vi "CheckForError-TMP.vi"(0 "Main Path":path) -> (1 "Array of Folders":path[](array[path]), 2 "PRAMMS-CommVRN":refnum<visa-resource-name>, 3 "Array of Files":path[](array[path]), 4 "Master Dir":path, 6 "Bundle-Meteo":T1={"cRIO address"="0.0.0.0", "Port Number"=0, "cRIO_commID"=refnum, "Cx"=FALSE}, 8 "This VI's Path":path, 10 "term":string, 11 "Go on ?":bool, 12 "Array of Baud Rates":u32[](array[numeric]), 13 "TCS-CommVRN":refnum<visa-resource-name>, 14 "Array of VISA refnum":refnum<visa-resource-name>[](array[refnum]), 15 "Serial":bool[](array[boolean]))   [LabVIEW 2011]
uses:
  Globals.vi
  <vilib>/Utility/config.llb/Read Key (U32).vi
  <vilib>/Utility/config.llb/Read Key (String).vi
  <vilib>/Instr/_visa.llb/VISA Configure Serial Port (Instr).vi
  <vilib>/Utility/config.llb/Read Key (Path).vi
  <vilib>/Utility/config.llb/NI_LVConfig.lvlib
panel:
  out "PRAMMS":bool
  out "ActiveDummy":bool
  out "TCS":bool
  out "TCP Error":errorcluster
  out "standard output":string
  out "standard error":string
  out "concatenated string":string
  out "Nettoyage":bool
  in  "restart":bool
  out "error out":errorcluster
  in  "cancel":bool
  in  "ignore":bool
  out "IDL":bool
  out "wget":bool
  out "Ports Series":bool
  out "SubVIs":bool
  out "config error out":errorcluster
  out "Camera":bool
  out "Starry Night":bool
  out "Configuration":bool
  out "Arborescence":bool
  # "Version sans GUI de ErrorCheck.vi  Vérifie :\n    - Existence des chemins/fichiers nécessaire\n    - Communication avec les différents périphériques\n    - Lien ActiveX avec Starry Night\n    - Vérifie la communication avec la station météo\n    - Vérifie l'état de la face avant des VIs utilisés\n    - Compatibilité des versions installées\n    - Vérifie la disponibilité des applications (wget, IDL)"
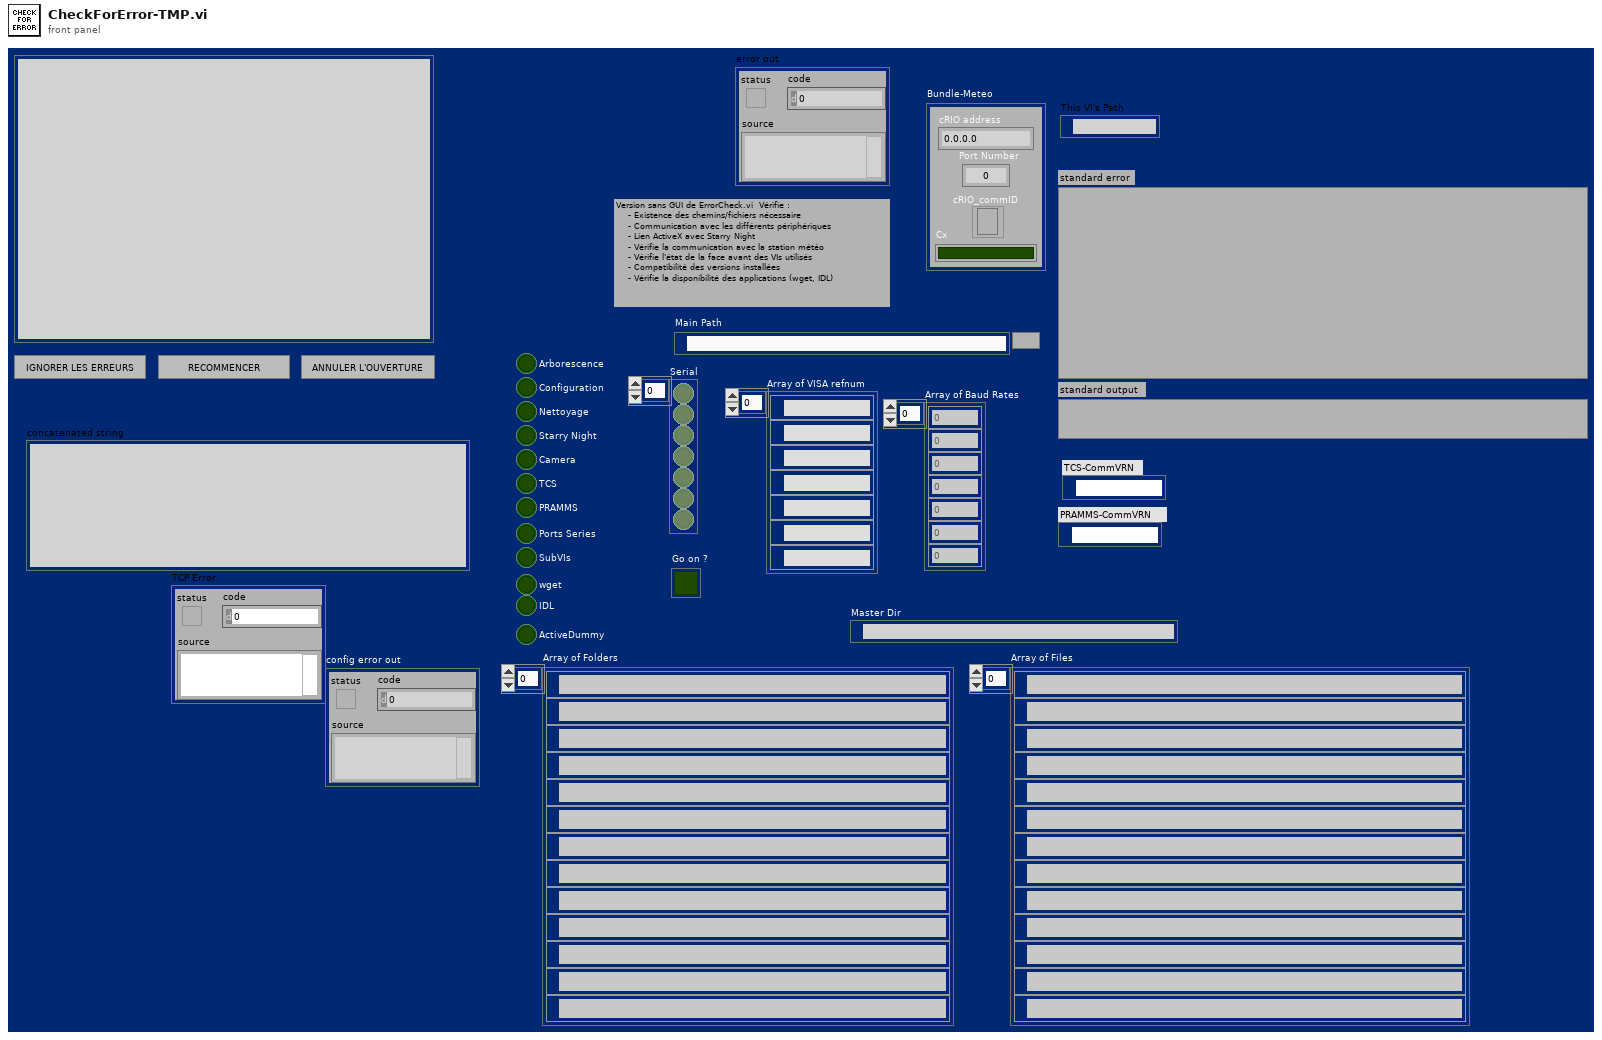
[diagram p1: front panel]
types:
  T1 = cluster{"cRIO address":string, "Port Number":u16, "cRIO_commID":refnum<k5>, "Cx":bool}
  T2 = enum8{"Enabled", "Disabled", "Disabled and Grayed Out"}
  T3 = typedef "NI_LVConfig.lvlib/Config Data RefNum.ctl" = refnum<k1>
  T4 = cluster{"value":string, u16, "connection ID":refnum<k5>, bool}
  T5 = enum16{"Left Button", "Center Button", "Right Button", "Window Close"}
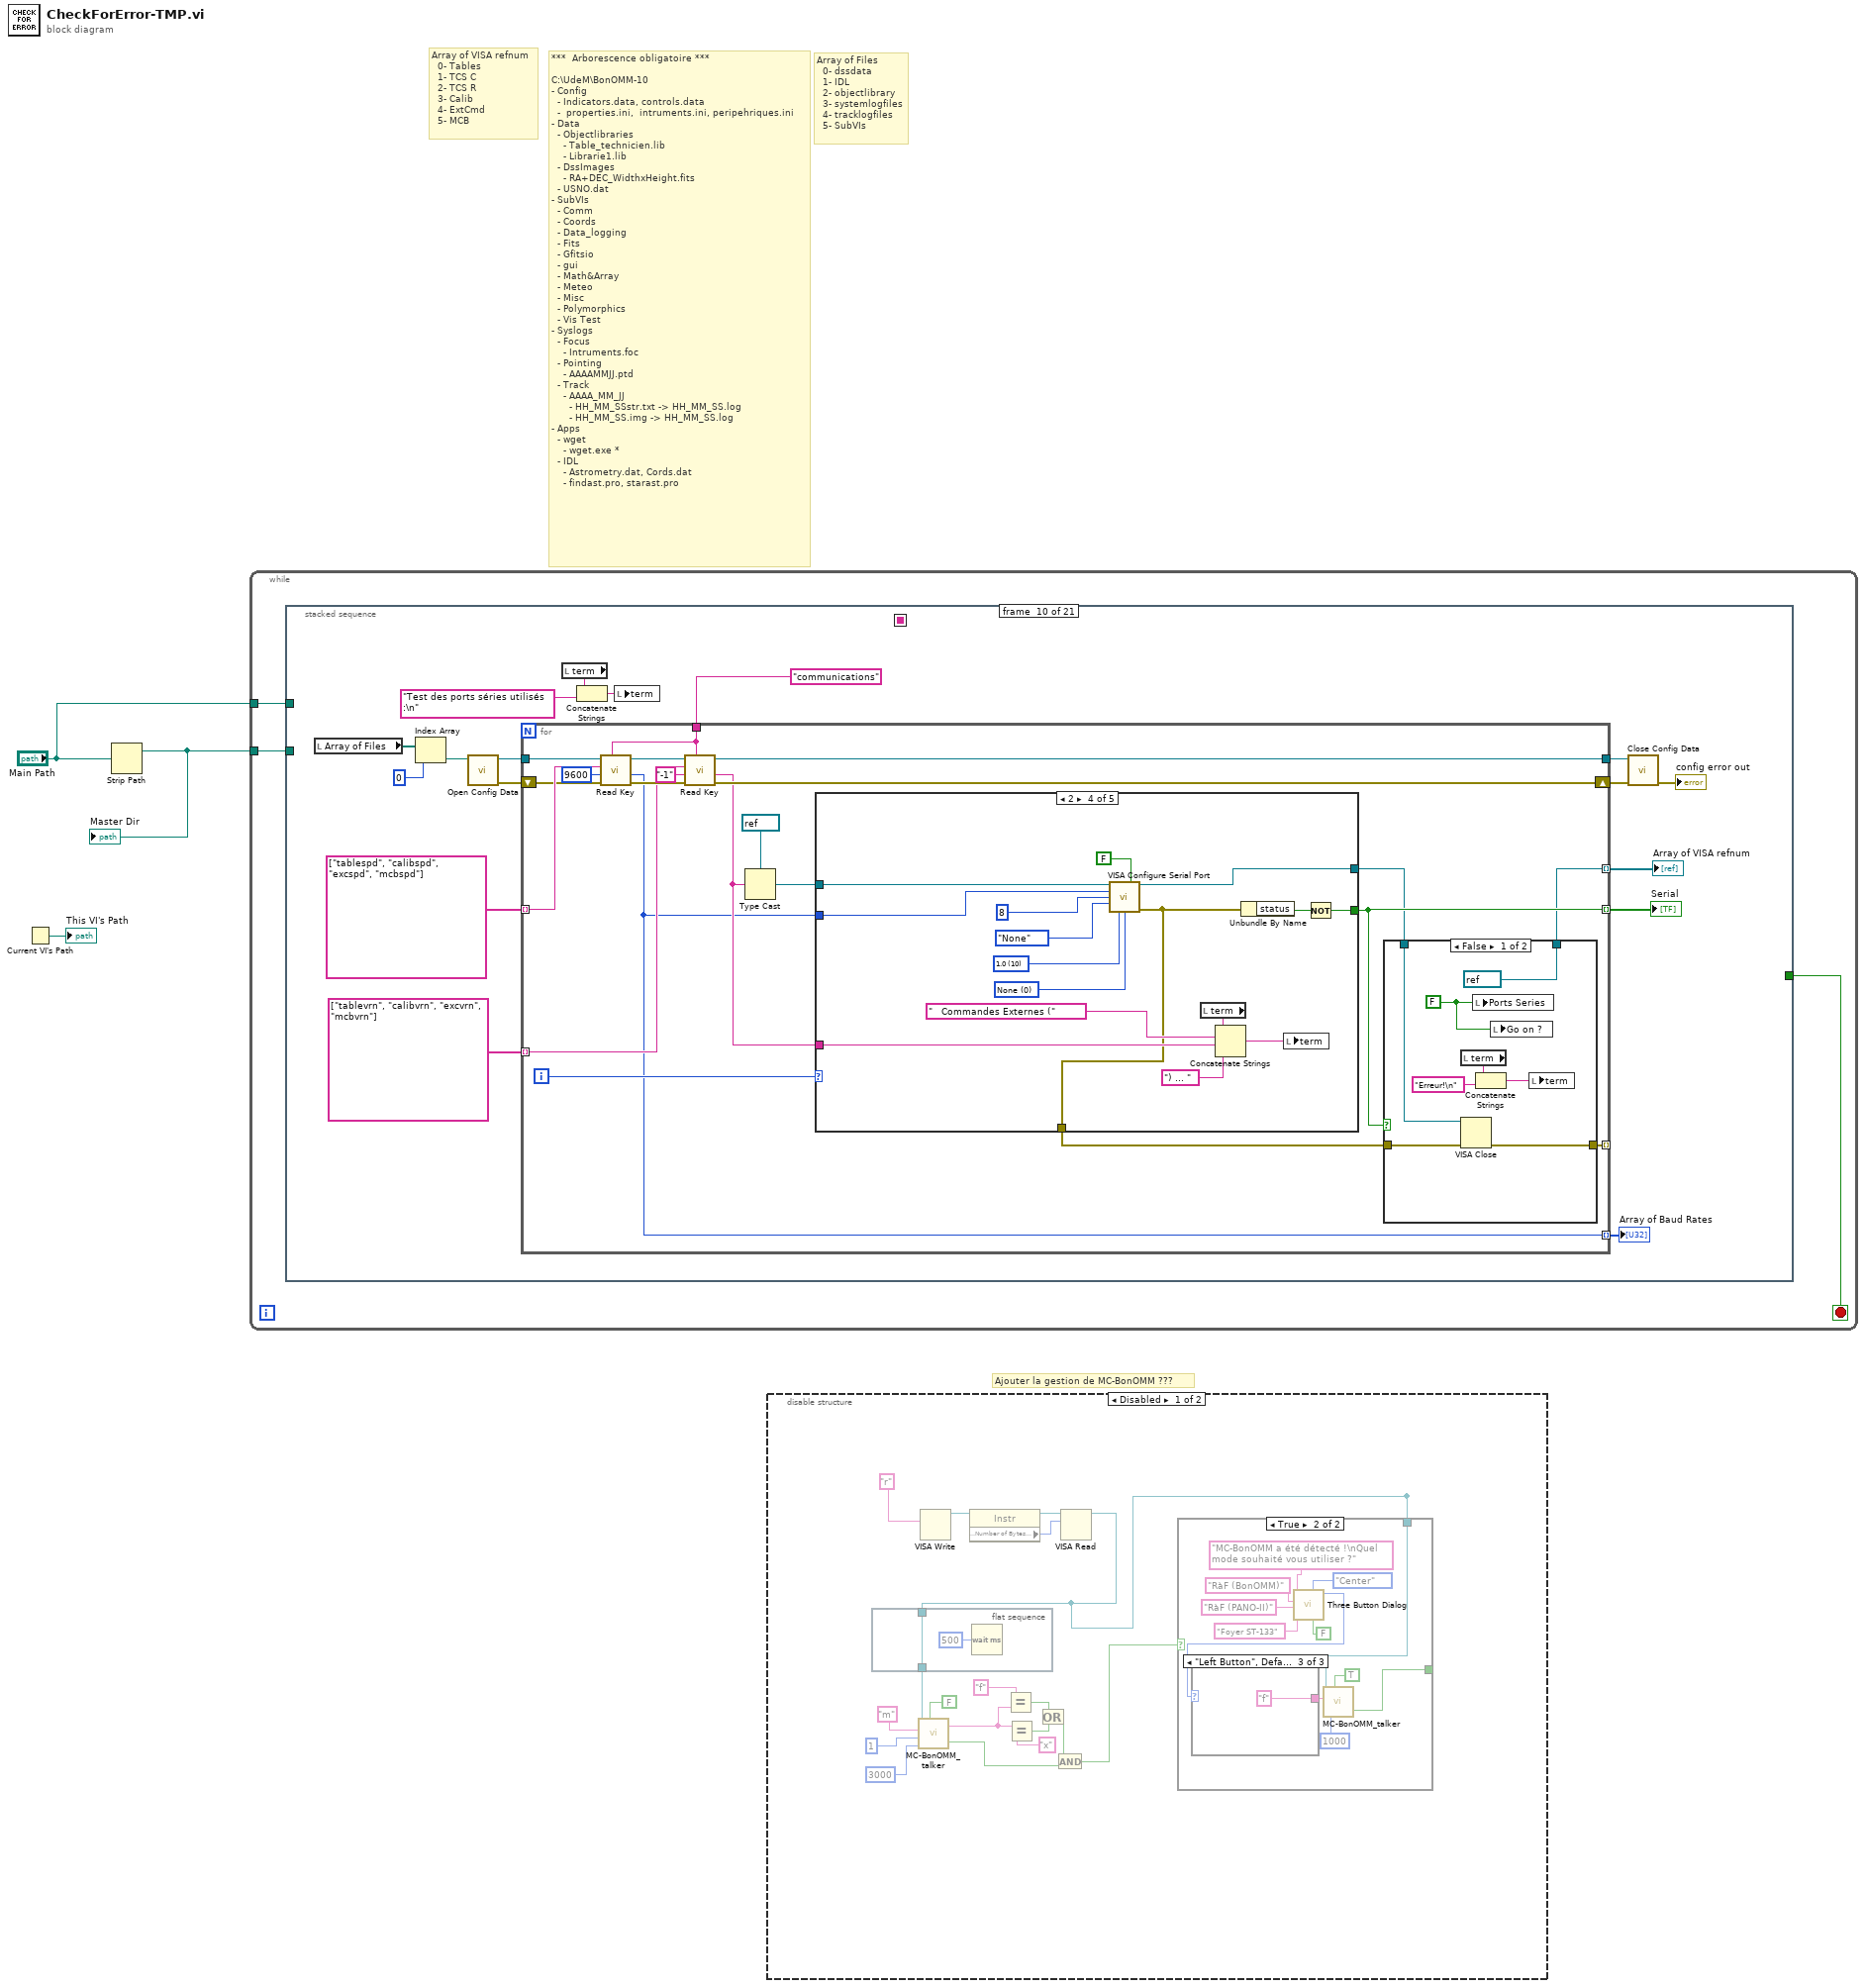
[diagram p0: block diagram]
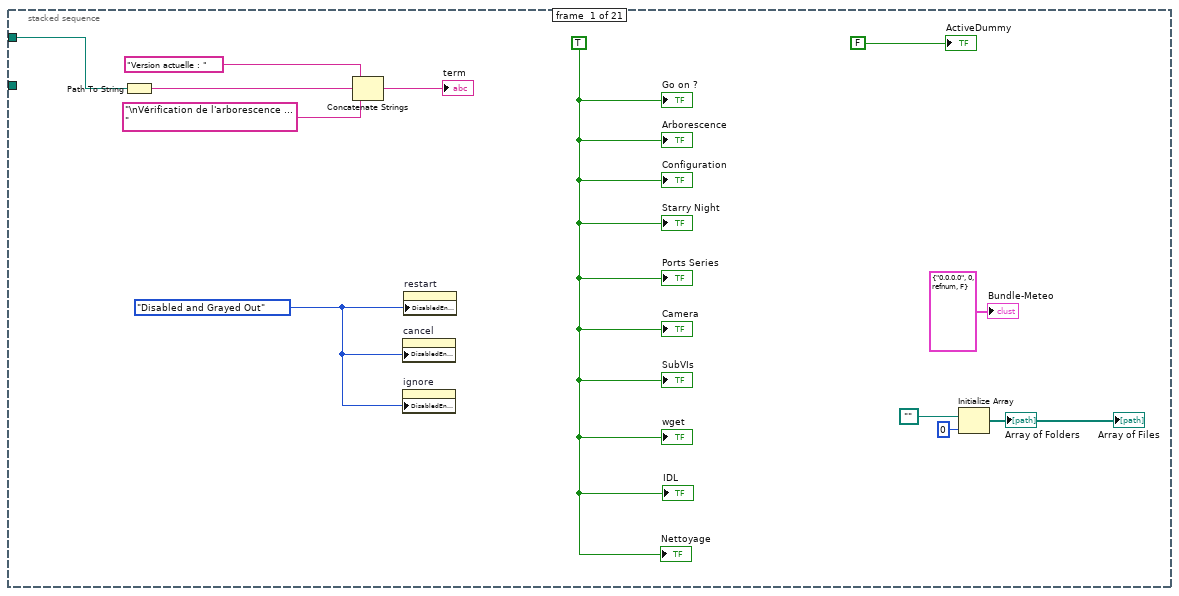
[diagram p2: hidden frame]
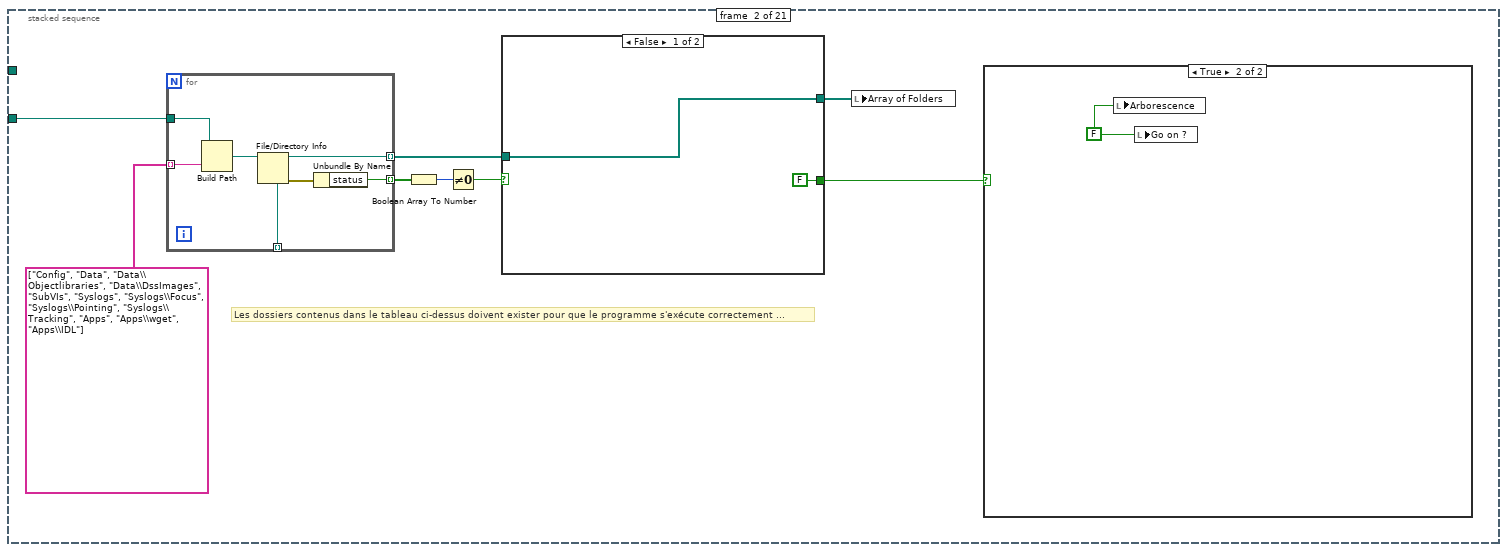
[diagram p3: hidden frame]
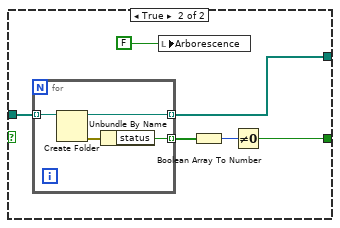
[diagram p5: hidden frame]
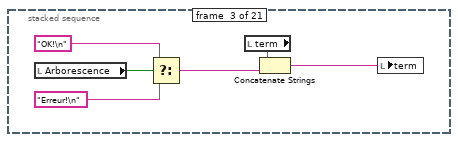
[diagram p6: hidden frame]
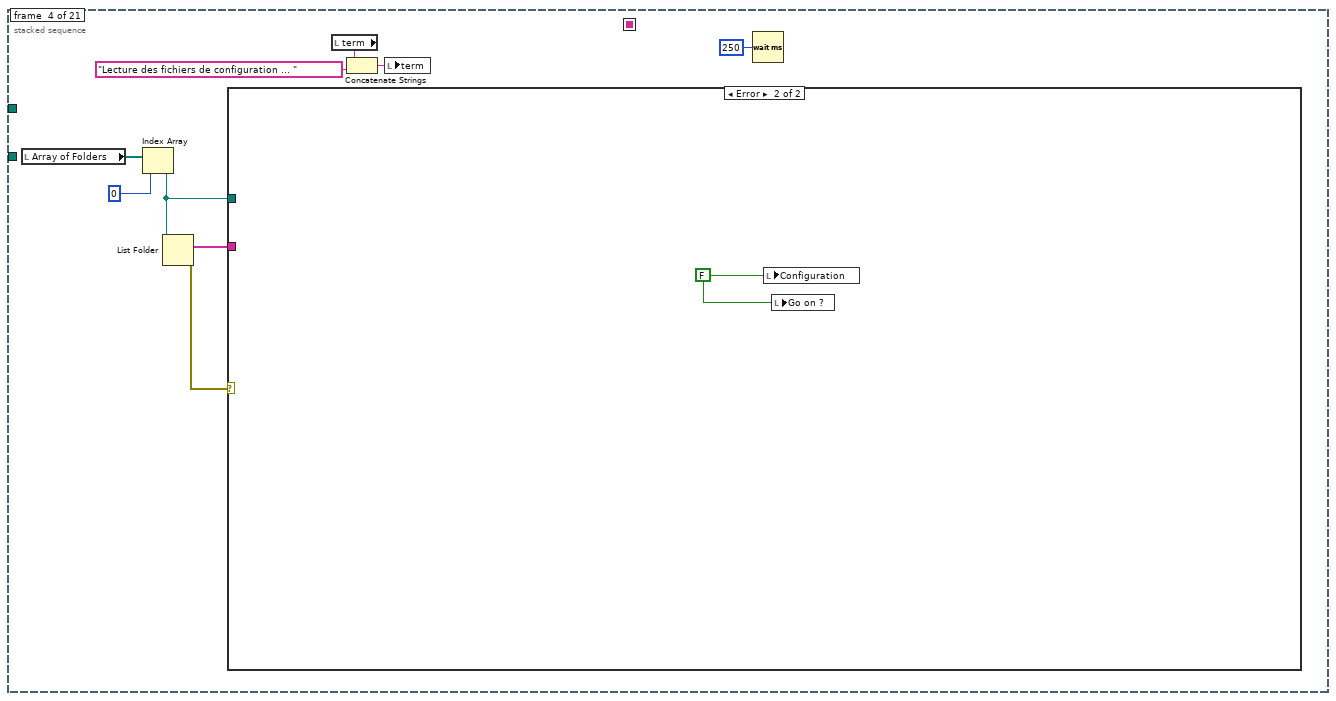
[diagram p7: hidden frame]
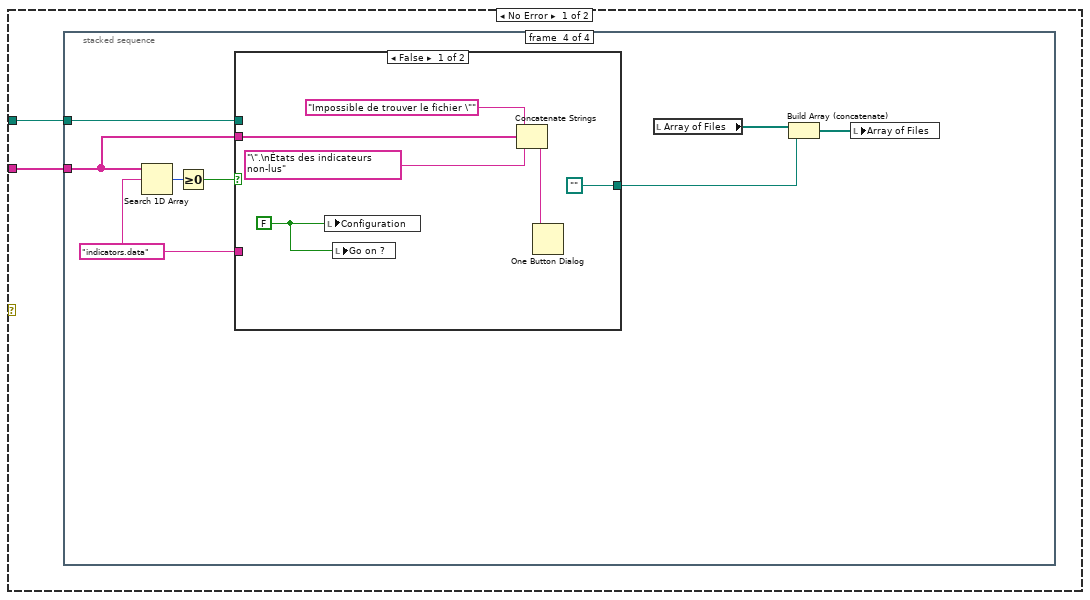
[diagram p8: hidden frame]
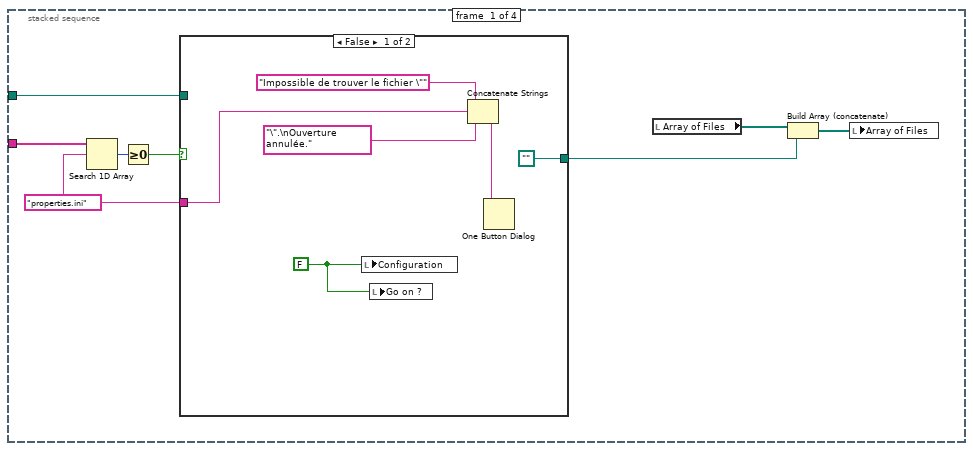
[diagram p9: hidden frame]
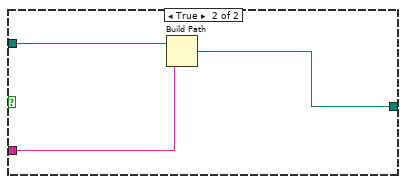
[diagram p10: hidden frame]
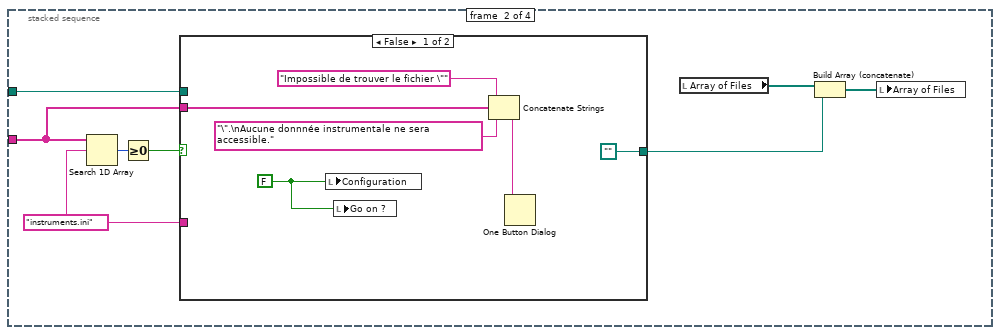
[diagram p11: hidden frame]
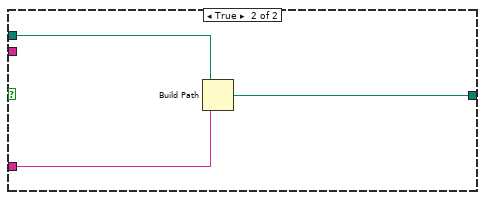
[diagram p12: hidden frame]
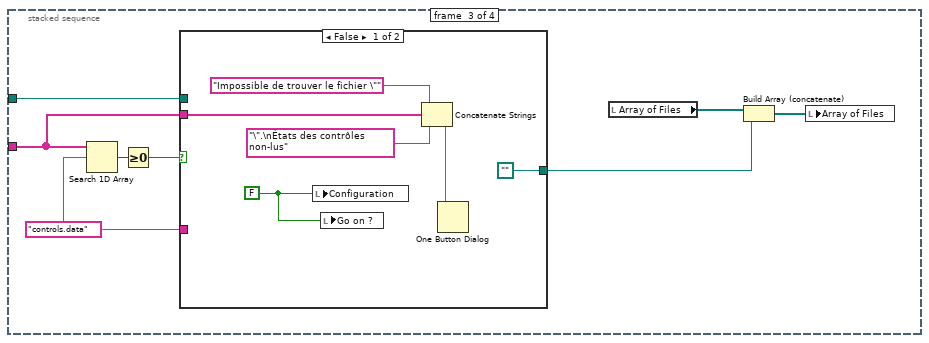
[diagram p13: hidden frame]
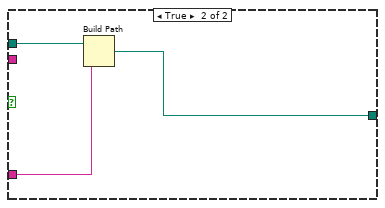
[diagram p14: hidden frame]
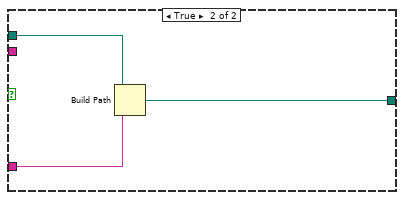
[diagram p15: hidden frame]
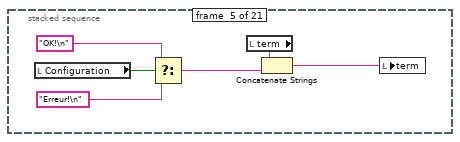
[diagram p16: hidden frame]
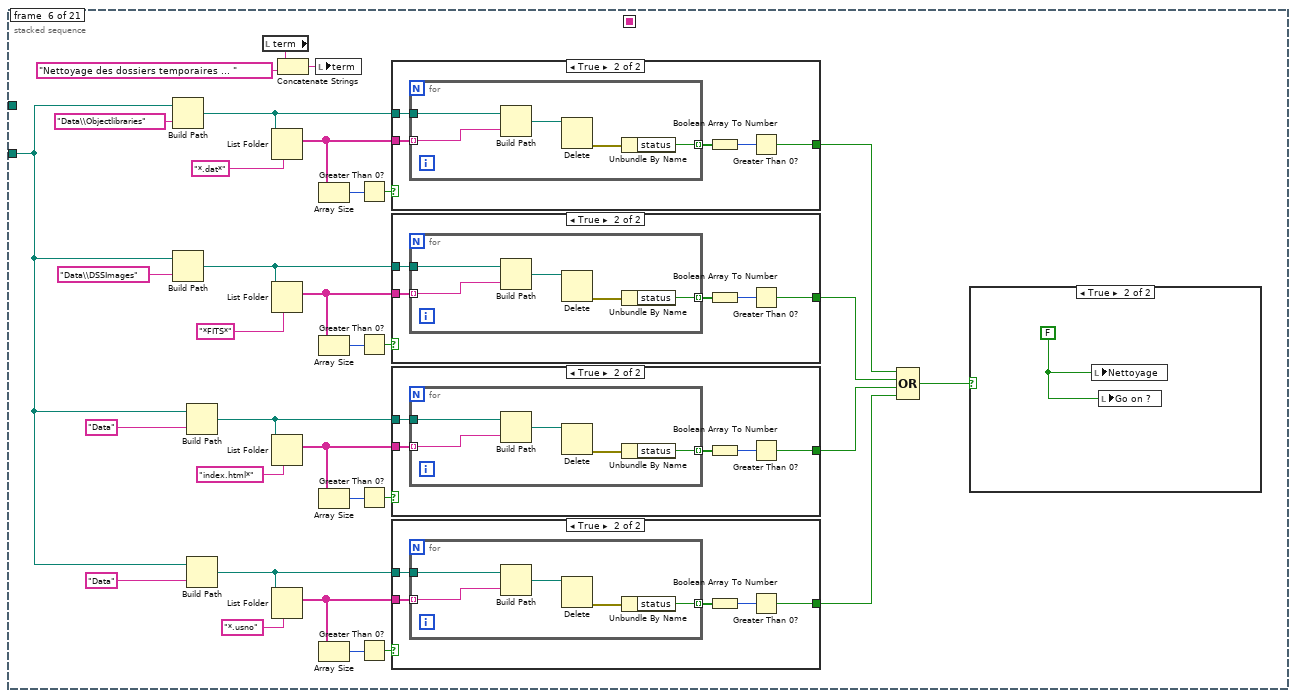
[diagram p17: hidden frame]
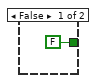
[diagram p18: hidden frame]
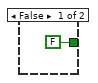
[diagram p19: hidden frame]
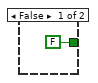
[diagram p20: hidden frame]
diagram:
  # "Array of Files\n  0- dssdata\n  1- IDL\n  2- objectlibrary\n  3- systemlogfiles\n  4- tracklogfiles\n  5- SubVIs"
  # "***  Arborescence obligatoire ***\n\nC:\\UdeM\\BonOMM-10\n-\tConfig\n  -\tIndicators.data, controls.data\n  -\t properties.ini,  intruments.ini, peripehriques.ini\n-\tData\n  -\tObjectlibraries\n    -\tTable_technicien.lib\n    -\tLibrarie1.lib\n  -\tDssImages\n    -\tRA+DEC_WidthxHeight.fits\n  -\tUSNO.dat\n-\tSubVIs\n  -\tComm\n  -\tCoords\n  -\tData_logging\n  -\tFits\n  -\tGfitsio\n  -\tgui\n  -\tMath&Array\n  -\tMeteo\n  -\tMisc\n  -\tPolymorphics\n  -\tVis Test\n-\tSyslogs\n  -\tFocus\n    -\tIntruments.foc\n  -\tPointing\n    -\tAAAAMMJJ.ptd\n  -\tTrack\n    -\tAAAA_MM_JJ\n      -\tHH_MM_SSstr.txt -> HH_MM_SS.log\n      -\tHH_MM_SS.img -> HH_MM_SS.log\n-\tApps\n  -\twget\n    -\twget.exe *\n  -\tIDL\n    -\tAstrometry.dat, Cords.dat\n    -\tfindast.pro, starast.pro"
  # "Array of VISA refnum\n  0- Tables\n  1- TCS C\n  2- TCS R\n  3- Calib\n  4- ExtCmd\n  5- MCB"
  # "Ajouter la gestion de MC-BonOMM ???"
  n1 = Current VI's Path() -> (path=→"This VI's Path":path)
  n2 = Strip Path(path="Main Path") -> (stripped path=w3:path)  [unwired: 1 out]
  "Master Dir" <- w3
  n3 = while {
    tunnel: w3 -> [w6]
    tunnel: "Main Path" -> [w5]
    stop <- w4 stop-if-true
    n4 = stacked-sequence {
      seq-local: [_ _ _ _ _ _ _ _ _ _ _ _ _ _ _ _ _ _ _ w594 _] -> [_ _ _ _ _ _ _ _ _ _ _ _ _ _ _ _ _ _ _ _ w630]
      tunnel: w6 -> [_ w25 _ _ _ w139 _ _ _ _ _ _ _ _ _ _ _ _ _ _ _]
      tunnel: w5 -> [w14 _ _ _ _ _ _ _ _ _ _ _ _ _ _ _ _ _ _ _ _]
      tunnel: [_ _ _ _ _ _ _ _ _ _ _ _ _ _ _ _ _ _ _ w595 _] -> w4
      frame #0 {
        w9 = T2."Disabled and Grayed Out" ("Disabled")
        w8 = TRUE ("Arborescence")
        n5 = Path To String(path=w14) -> (string=w18:string)
        n6 = Concatenate Strings("Version actuelle : ", w18, "\nVérification de l'arborescence ... ") -> (→"term":string)
        n7 = property on="cancel" class="Bool"("DisabledEnum"=w9) -> ()  [unwired: 2 in, 2 out]
        n8 = property on="ignore" class="Bool"("DisabledEnum"=w9) -> ()  [unwired: 2 in, 2 out]
        n9 = property on="restart" class="Bool"("DisabledEnum"=w9) -> ()  [unwired: 2 in, 2 out]
        n10 = Initialize Array(path "" ("path dup"), 0 ("dimension size")) -> (→"Array of Folders" →"Array of Files":path[])
        "Arborescence" <- w8
        "Go on ?" <- w8
        "Configuration" <- w8
        "Starry Night" <- w8
        "Camera" <- w8
        "SubVIs" <- w8
        "Ports Series" <- w8
        "wget" <- w8
        "IDL" <- w8
        "Bundle-Meteo" <- T1 {"cRIO address"="0.0.0.0", "Port Number"=0, "cRIO_commID"=refnum, "Cx"=FALSE} ("Bundle-Meteo")
        "Nettoyage" <- w8
        "ActiveDummy" <- FALSE ("Arborescence")
      }
      frame #1 {
        # "Les dossiers contenus dans le tableau ci-dessus doivent exister pour que le programme s'exécute correctement ..."
        n11 = for {
          tunnel: string[] ["Config", "Data", "Data\\Objectlibraries", "Data\\DssImages", "SubVIs", "Syslogs", "Syslogs\\Focus", "Syslogs\\Pointing", "Syslogs\\Tracking", "Apps", "Apps\\wget", "Apps\\IDL"] -> [w45] mode=indexing
          tunnel: w25 -> [w46]
          tunnel: [w43] -> w21 mode=indexing
          tunnel: [w42] -> _ mode=indexing
          tunnel: [w40] -> w24 mode=indexing
          n12 = Build Path(base path=w46, name or relative path=w45) -> (appended path=w44:path)
          n13 = File/Directory Info(path=w44) -> (path out=w43:path, error out=w41:errorcluster, resolved path=w42:path)  [unwired: 1 in, 4 out]
          n14 = Unbundle By Name(w41) -> ("status"=w40:bool)
        }
        n15 = Boolean Array To Number(Boolean array=w24) -> (number=w23:u32)
        n16 = Not Equal To 0?(x=w23) -> (x != 0?=w22:bool)
        n17 = case shown="False" w22 {
          tunnel: w21 -> [w28 w35]
          tunnel: [FALSE w32] -> w20
          tunnel: [w28 w31] -> w19
          frame False {
          }
          frame True {
            n18 = for {
              tunnel: w35 -> [w39] mode=indexing
              tunnel: [w37] -> w33 mode=indexing
              tunnel: [w36] -> w31 mode=indexing
              n19 = Create Folder(path (use dialog)=w39) -> (created path=w36:path, error out=w38:errorcluster)  [unwired: 2 in, 1 out]
              n20 = Unbundle By Name(w38) -> ("status"=w37:bool)
            }
            n21 = local write "Arborescence"(FALSE) -> ()
            n22 = Boolean Array To Number(Boolean array=w33) -> (number=w34:u32)
            n23 = Not Equal To 0?(x=w34) -> (x != 0?=w32:bool)
          }
        }
        n24 = local write "Array of Folders"(w19) -> ()
        n25 = case shown="True" w20 {
          frame False {
          }
          frame True {
            w27 = FALSE
            n26 = local write "Arborescence"(w27) -> ()
            n27 = local write "Go on ?"(w27) -> ()
          }
        }
      }
      frame #2 {
        n28 = local read "Arborescence"() -> (w49:bool)
        n29 = Select(t="OK!\n" ("string"), s=w49, f="Erreur!\n" ("string")) -> (s? t:f=w50:string)
        n30 = local read "term"() -> (w51:string)
        n31 = Concatenate Strings(w51, w50) -> (w52:string)
        n32 = local write "term"(w52) -> ()
      }
      frame #3 {
        n33 = local read "Array of Folders"() -> (w55:path[])
        n34 = Index Array(array=w55, index=0) -> (element=w53:path)
        n35 = List Folder(path=w53) -> (filenames=w58:string[], error out=w56:errorcluster)  [unwired: 3 in, 2 out]
        n36 = case shown="Error" w56 {
          tunnel: w58 -> [w63 _]
          tunnel: w53 -> [w62 _]
          frame No Error {
            n37 = stacked-sequence {
              tunnel: w63 -> [w69 w86 w103 w120]
              tunnel: w62 -> [w66 w84 w102 w119]
              frame #0 {
                w65 = "properties.ini"
                n38 = Search 1D Array(1D array=w69, element=w65) -> (index of element=w71:i32)  [unwired: 1 in]
                n39 = Greater Or Equal To 0?(x=w71) -> (x >= 0?=w70:bool)
                n40 = case shown="False" w70 {
                  tunnel: w66 -> [_ w80]
                  tunnel: w65 -> [w73 w79]
                  tunnel: [path "" w78] -> w64
                  frame False {
                    w74 = FALSE ("Configuration")
                    n41 = local write "Configuration"(w74) -> ()
                    n42 = local write "Go on ?"(w74) -> ()
                    n43 = Concatenate Strings("Impossible de trouver le fichier \"", w73, "\".\nOuverture annulée.") -> (w75:string)
                    n44 = One Button Dialog(message=w75) -> ()  [unwired: 1 in, 1 out]
                  }
                  frame True {
                    n45 = Build Path(base path=w80, name or relative path=w79) -> (appended path=w78:path)
                  }
                }
                n46 = local read "Array of Files"() -> (w68:path[])
                n47 = Build Array (concatenate)(w68, w64) -> (w67:path[])
                n48 = local write "Array of Files"(w67) -> ()
              }
              frame #1 {
                w85 = "instruments.ini"
                n49 = Search 1D Array(1D array=w86, element=w85) -> (index of element=w88:i32)  [unwired: 1 in]
                n50 = Greater Or Equal To 0?(x=w88) -> (x >= 0?=w87:bool)
                n51 = case shown="False" w87 {
                  tunnel: w86 -> [w92 _]
                  tunnel: w85 -> [_ w97]
                  tunnel: w84 -> [_ w96]
                  tunnel: [path "" w95] -> w81
                  frame False {
                    w90 = FALSE ("Configuration")
                    n52 = local write "Configuration"(w90) -> ()
                    n53 = local write "Go on ?"(w90) -> ()
                    n54 = Concatenate Strings("Impossible de trouver le fichier \"", w92, "\".\nAucune donnnée instrumentale ne sera accessible.") -> (w91:string)
                    n55 = One Button Dialog(message=w91) -> ()  [unwired: 1 in, 1 out]
                  }
                  frame True {
                    n56 = Build Path(base path=w96, name or relative path=w97) -> (appended path=w95:path)
                  }
                }
                n57 = local read "Array of Files"() -> (w83:path[])
                n58 = Build Array (concatenate)(w83, w81) -> (w82:path[])
                n59 = local write "Array of Files"(w82) -> ()
              }
              frame #2 {
                w101 = "controls.data"
                n60 = Search 1D Array(1D array=w103, element=w101) -> (index of element=w105:i32)  [unwired: 1 in]
                n61 = Greater Or Equal To 0?(x=w105) -> (x >= 0?=w104:bool)
                n62 = case shown="False" w104 {
                  tunnel: w103 -> [w109 _]
                  tunnel: w102 -> [_ w114]
                  tunnel: w101 -> [_ w113]
                  tunnel: [path "" w112] -> w98
                  frame False {
                    w107 = FALSE ("Configuration")
                    n63 = local write "Configuration"(w107) -> ()
                    n64 = local write "Go on ?"(w107) -> ()
                    n65 = Concatenate Strings("Impossible de trouver le fichier \"", w109, "\".\nÉtats des contrôles non-lus") -> (w108:string)
                    n66 = One Button Dialog(message=w108) -> ()  [unwired: 1 in, 1 out]
                  }
                  frame True {
                    n67 = Build Path(base path=w114, name or relative path=w113) -> (appended path=w112:path)
                  }
                }
                n68 = local read "Array of Files"() -> (w100:path[])
                n69 = Build Array (concatenate)(w100, w98) -> (w99:path[])
                n70 = local write "Array of Files"(w99) -> ()
              }
              frame #3 {
                w118 = "indicators.data"
                n71 = Search 1D Array(1D array=w120, element=w118) -> (index of element=w122:i32)  [unwired: 1 in]
                n72 = Greater Or Equal To 0?(x=w122) -> (x >= 0?=w121:bool)
                n73 = case shown="False" w121 {
                  tunnel: w120 -> [w126 _]
                  tunnel: w119 -> [_ w131]
                  tunnel: w118 -> [_ w130]
                  tunnel: [path "" w129] -> w115
                  frame False {
                    w124 = FALSE ("Configuration")
                    n74 = local write "Configuration"(w124) -> ()
                    n75 = local write "Go on ?"(w124) -> ()
                    n76 = Concatenate Strings("Impossible de trouver le fichier \"", w126, "\".\nÉtats des indicateurs non-lus") -> (w125:string)
                    n77 = One Button Dialog(message=w125) -> ()  [unwired: 1 in, 1 out]
                  }
                  frame True {
                    n78 = Build Path(base path=w131, name or relative path=w130) -> (appended path=w129:path)
                  }
                }
                n79 = local read "Array of Files"() -> (w117:path[])
                n80 = Build Array (concatenate)(w117, w115) -> (w116:path[])
                n81 = local write "Array of Files"(w116) -> ()
              }
            }
          }
          frame Error {
            w132 = FALSE ("Configuration")
            n82 = local write "Configuration"(w132) -> ()
            n83 = local write "Go on ?"(w132) -> ()
          }
        }
        n84 = local read "term"() -> (w60:string)
        n85 = Concatenate Strings(w60, "Lecture des fichiers de configuration ... " ("string")) -> (w61:string)
        n86 = local write "term"(w61) -> ()
        n87 = Wait (ms)(milliseconds to wait=u32 250) -> ()  [unwired: 1 out]
      }
      frame #4 {
        n88 = local read "Configuration"() -> (w135:bool)
        n89 = Select(t="OK!\n" ("string"), s=w135, f="Erreur!\n" ("string")) -> (s? t:f=w136:string)
        n90 = local read "term"() -> (w137:string)
        n91 = Concatenate Strings(w137, w136) -> (w138:string)
        n92 = local write "term"(w138) -> ()
      }
      frame #5 {
        n93 = Build Path(base path=w139, name or relative path="Data\\Objectlibraries") -> (appended path=w164:path)
        n94 = Build Path(base path=w139, name or relative path="Data\\DSSImages") -> (appended path=w162:path)
        n95 = Build Path(base path=w139, name or relative path="Data") -> (appended path=w148:path)
        n96 = Build Path(base path=w139, name or relative path="Data") -> (appended path=w145:path)
        n97 = local read "term"() -> (w170:string)
        n98 = List Folder(path=w164, pattern="*.dat*") -> (filenames=w166:string[])  [unwired: 2 in, 3 out]
        n99 = List Folder(path=w162, pattern="*FITS*") -> (filenames=w160:string[])  [unwired: 2 in, 3 out]
        n100 = List Folder(path=w148, pattern="index.html*") -> (filenames=w150:string[])  [unwired: 2 in, 3 out]
        n101 = List Folder(path=w145, pattern="*.usno") -> (filenames=w144:string[])  [unwired: 2 in, 3 out]
        n102 = Concatenate Strings(w170, "Nettoyage des dossiers temporaires ... " ("string")) -> (w171:string)
        n103 = local write "term"(w171) -> ()
        n104 = Array Size(array=w166) -> (size(s)=w167:i32)
        n105 = Array Size(array=w160) -> (size(s)=w159:i32)
        n106 = Array Size(array=w150) -> (size(s)=w151:i32)
        n107 = Array Size(array=w144) -> (size(s)=w143:i32)
        n108 = Greater Than 0?(x=w167) -> (x > 0?=w168:bool)
        n109 = Greater Than 0?(x=w159) -> (x > 0?=w158:bool)
        n110 = Greater Than 0?(x=w151) -> (x > 0?=w152:bool)
        n111 = Greater Than 0?(x=w143) -> (x > 0?=w142:bool)
        n112 = case shown="True" w168 {
          tunnel: w166 -> [_ w210]
          tunnel: w164 -> [_ w209]
          tunnel: [FALSE w206] -> w156
          frame False {
          }
          frame True {
            n113 = for {
              tunnel: w210 -> [w214] mode=indexing
              tunnel: w209 -> [w215]
              tunnel: [w211] -> w208 mode=indexing
              n114 = Build Path(base path=w215, name or relative path=w214) -> (appended path=w213:path)
              n115 = Delete(path (use dialog)=w213) -> (error out=w212:errorcluster)  [unwired: 4 in, 2 out]
              n116 = Unbundle By Name(w212) -> ("status"=w211:bool)
            }
            n117 = Boolean Array To Number(Boolean array=w208) -> (number=w207:u32)
            n118 = Greater Than 0?(x=w207) -> (x > 0?=w206:bool)
          }
        }
        n119 = case shown="True" w158 {
          tunnel: w160 -> [_ w199]
          tunnel: w162 -> [_ w198]
          tunnel: [FALSE w195] -> w155
          frame False {
          }
          frame True {
            n120 = for {
              tunnel: w199 -> [w203] mode=indexing
              tunnel: w198 -> [w204]
              tunnel: [w200] -> w197 mode=indexing
              n121 = Build Path(base path=w204, name or relative path=w203) -> (appended path=w202:path)
              n122 = Delete(path (use dialog)=w202) -> (error out=w201:errorcluster)  [unwired: 4 in, 2 out]
              n123 = Unbundle By Name(w201) -> ("status"=w200:bool)
            }
            n124 = Boolean Array To Number(Boolean array=w197) -> (number=w196:u32)
            n125 = Greater Than 0?(x=w196) -> (x > 0?=w195:bool)
          }
        }
        n126 = case shown="True" w152 {
          tunnel: w150 -> [_ w188]
          tunnel: w148 -> [_ w187]
          tunnel: [FALSE w184] -> w149
          frame False {
          }
          frame True {
            n127 = for {
              tunnel: w188 -> [w192] mode=indexing
              tunnel: w187 -> [w193]
              tunnel: [w189] -> w186 mode=indexing
              n128 = Build Path(base path=w193, name or relative path=w192) -> (appended path=w191:path)
              n129 = Delete(path (use dialog)=w191) -> (error out=w190:errorcluster)  [unwired: 4 in, 2 out]
              n130 = Unbundle By Name(w190) -> ("status"=w189:bool)
            }
            n131 = Boolean Array To Number(Boolean array=w186) -> (number=w185:u32)
            n132 = Greater Than 0?(x=w185) -> (x > 0?=w184:bool)
          }
        }
        n133 = case shown="True" w142 {
          tunnel: w144 -> [_ w177]
          tunnel: w145 -> [_ w176]
          tunnel: [FALSE w173] -> w140
          frame False {
          }
          frame True {
            n134 = for {
              tunnel: w177 -> [w181] mode=indexing
              tunnel: w176 -> [w182]
              tunnel: [w178] -> w175 mode=indexing
              n135 = Build Path(base path=w182, name or relative path=w181) -> (appended path=w180:path)
              n136 = Delete(path (use dialog)=w180) -> (error out=w179:errorcluster)  [unwired: 4 in, 2 out]
              n137 = Unbundle By Name(w179) -> ("status"=w178:bool)
            }
            n138 = Boolean Array To Number(Boolean array=w175) -> (number=w174:u32)
            n139 = Greater Than 0?(x=w174) -> (x > 0?=w173:bool)
          }
        }
        n140 = Compound Arithmetic op=OR(w156, w155, w149, w140) -> (w157:bool)
        n141 = case shown="True" w157 {
          frame False {
          }
          frame True {
            w216 = FALSE
            n142 = local write "Nettoyage"(w216) -> ()
            n143 = local write "Go on ?"(w216) -> ()
          }
        }
      }
      frame #6 {
        n144 = local read "Nettoyage"() -> (w219:bool)
        n145 = Select(t="OK!\n" ("string"), s=w219, f="Erreur!\n" ("string")) -> (s? t:f=w220:string)
        n146 = local read "term"() -> (w221:string)
        n147 = Concatenate Strings(w221, w220) -> (w222:string)
        n148 = local write "term"(w222) -> ()
      }
      frame #7 {
        n149 = local read "term"() -> (w229:string)
        n150 = Concatenate Strings(w229, "Test du lien ActiveX avec Starry Night ... " ("string")) -> (w230:string)
        n151 = local write "term"(w230) -> ()
        n152 = Automation Open(Automation Refnum=refnum<k7> refnum ("ScopeSim._Telescope")) -> (Automation Refnum=w223:refnum<k7>, error out=w226:errorcluster)  [unwired: 3 in]
        n153 = Unbundle By Name(w226) -> ("status"=w225:bool)
        n154 = case shown="True" w225 {
          tunnel: w223 -> [w233 _]
          tunnel: [w232 FALSE ("Connected")] -> w227
          frame False {
            n155 = property class="_Telescope"(reference=w233) -> (reference out=w231:refnum<k7>, "Connected"=w232:bool)  [unwired: 1 in, 1 out]
            n156 = Close Reference(reference=w231) -> ()  [unwired: 1 in, 1 out]
          }
          frame True {
          }
        }
        n157 = global write "Globals.vi" "ScopeSim._Telescope"(w223) -> ()
        n158 = case shown="True" w227 {
          frame False {
            w235 = FALSE
            n159 = local write "Starry Night"(w235) -> ()
            n160 = local write "Go on ?"(w235) -> ()
          }
          frame True {
          }
        }
      }
      frame #8 {
        n161 = local read "Starry Night"() -> (w236:bool)
        n162 = Select(t="OK!\n" ("string"), s=w236, f="Erreur!\n" ("string")) -> (s? t:f=w239:string)
        n163 = local read "term"() -> (w240:string)
        n164 = Concatenate Strings(w240, w239) -> (w241:string)
        n165 = local write "term"(w241) -> ()
      }
      frame #9 {
        n166 = local read "Array of Files"() -> (w244:path[])
        n167 = Index Array(array=w244, index=0) -> (element=w243:path)
        n168 = call <vilib>:"Open Config Data.vi"("configuration file path"=w243) -> ("error out"=w252:errorcluster, "refnum"=w254:T3)  [unwired: 8 in, 1 out]
        n169 = for {
          tunnel: string[] ["tablespd", "calibspd", "excspd", "mcbspd"] -> [w275] mode=indexing
          tunnel: string[] ["tablevrn", "calibvrn", "excvrn", "mcbvrn"] -> [w274] mode=indexing
          tunnel: "communications" -> [w267]
          tunnel: w254 -> [w277]
          tunnel: [w276] -> w253
          shift-right: [w272] -> w251
          shift-left: w252 -> [w273]
          tunnel: [w264] -> w247 mode=indexing
          tunnel: [w266] -> w246 mode=indexing
          tunnel: [w260] -> w245 mode=indexing
          tunnel: [w262] -> _ mode=indexing
          i -> [w268]
          n170 = call-poly <vilib>:"Read Key.vi"("section"=w267, "error in (no error)"=w273, "default value"=u32 9600, "key"=w275, "refnum"=w277) -> ("error out"=w278:errorcluster, "value"=w260:u32, "refnum out"=w279:T3)  [unwired: 3 in, 1 out]
          n171 = call-poly <vilib>:"Read Key.vi"("section"=w267, "error in (no error)"=w278, "default value"="-1", "key"=w274, "refnum"=w279) -> ("error out"=w272:errorcluster, "value"=w263:string, "refnum out"=w276:T3)  [unwired: 3 in, 1 out]
          n172 = Type Cast(type=refnum<visa-resource-name> "-1" ("Table VRN"), x=w263) -> (*(type *) &x=w261:refnum<visa-resource-name>)
          n173 = case shown="2" w268 {
            tunnel: w261 -> [_ w308 w317 w338 w354]
            tunnel: [refnum<visa-resource-name> "-1" ("Table VRN") w300 w329 w336 w352] -> w265
            tunnel: [FALSE ("ok ?") w304 w330 w348 w359] -> w266
            tunnel: w263 -> [_ w312 w324 w343 w360]
            tunnel: w260 -> [_ w302 w319 w337 w353]
            tunnel: [errorcluster {"status"=FALSE, "code"=0, "source"=""} ("error out") w297 w316 w335 w351] -> w259
            frame -1, Default {
              (unwired) "Bizzarerie ... " ("string")
            }
            frame 0 {
              n174 = control-ref of="ActiveDummy"() -> (w296:refnum<vi>)
              n175 = Equal?(x=refnum<visa-resource-name> "N/A" ("Table VRN"), y=w308) -> (x = y?=w306:bool)
              n176 = Select(t=refnum<visa-resource-name> "-1", s=w306, f=w308) -> (s? t:f=w303:refnum<visa-resource-name>)
              n177 = call "Newmark-Initialize.vi"("VISA resource name"=w303, "ActiveStages"=string[] ["AX", "AY", "AZ"], "baud rate"=w302, "Timeout"=u32 1000, "Bool Refnum"=w296) -> ("VISA resource name out"=w300:refnum<visa-resource-name>, "Error?"=w299:bool, "Error OUT"=w297:errorcluster)  [unwired: 8 in]
              n178 = Not(x=w306) -> (.not. x?=w307:bool)
              n179 = local read "term"() -> (w315:string)
              n180 = Concatenate Strings(w315, "   Table de guidage (" ("string"), w312, ") ... " ("string")) -> (w314:string)
              n181 = And(x=w299, y=w307) -> (x .and. y?=w305:bool)
              n182 = Not(x=w305) -> (.not. x?=w304:bool)
              n183 = local write "term"(w314) -> ()
            }
            frame 1 {
              w323 = u16 0 items=["None", "XON/XOFF", "RTS/CTS", "XON/XOFF & RTS/CTS", "DTR/DSR", "XON/XOFF & DTR/DSR"] ("flow control (0:none)")
              w322 = u16 10 items=["1.0"=10, "1.5"=15, "2.0"=20] ("stop bits (10: 1 bit)")
              n184 = call-poly "VISA Configure Serial Port"("VISA resource name"=w317, "baud rate (9600)"=w319, "data bits (8)"=u16 8, "parity (0:none)"=enum16{"None", "Odd", "Even", "Mark", "Space"}."None", "stop bits (10: 1 bit)"=w322, "flow control (0:none)"=w323) -> ("VISA resource name out"=w318:refnum<visa-resource-name>, "error out"=w316:errorcluster)  [unwired: 8 in]
              n185 = call "Controle_des_lampe.vi"("VISA resource name"=w318, "Status In"=bool[] [FALSE, FALSE, FALSE]) -> ("VISA resource name dup"=w329:refnum<visa-resource-name>, "Status Out"=w333:bool[])  [unwired: 1 out]
              n186 = local read "term"() -> (w328:string)
              n187 = Concatenate Strings(w328, "   Module de caibration (" ("string"), w324, ") ... " ("string")) -> (w327:string)
              n188 = Boolean Array To Number(Boolean array=w333) -> (number=w331:u32)
              n189 = Equal To 0?(x=w331) -> (x = 0?=w330:bool)
              n190 = local write "term"(w327) -> ()
            }
            frame 2 {
              w342 = u16 0 items=["None", "XON/XOFF", "RTS/CTS", "XON/XOFF & RTS/CTS", "DTR/DSR", "XON/XOFF & DTR/DSR"] ("flow control (0:none)")
              w341 = u16 10 items=["1.0"=10, "1.5"=15, "2.0"=20] ("stop bits (10: 1 bit)")
              n191 = call-poly "VISA Configure Serial Port"("VISA resource name"=w338, "Enable Termination\nChar (T)"=FALSE ("Enable Termination\nChar (T)"), "baud rate (9600)"=w337, "data bits (8)"=u16 8, "parity (0:none)"=enum16{"None", "Odd", "Even", "Mark", "Space"}."None", "stop bits (10: 1 bit)"=w341, "flow control (0:none)"=w342) -> ("VISA resource name out"=w336:refnum<visa-resource-name>, "error out"=w335:errorcluster)  [unwired: 7 in]
              n192 = local read "term"() -> (w347:string)
              n193 = Concatenate Strings(w347, "   Commandes Externes (" ("string"), w343, ") ... " ("string")) -> (w346:string)
              n194 = Unbundle By Name(w335) -> ("status"=w349:bool)
              n195 = local write "term"(w346) -> ()
              n196 = Not(x=w349) -> (.not. x?=w348:bool)
            }
            frame 3 {
              w358 = u16 0 items=["None", "XON/XOFF", "RTS/CTS", "XON/XOFF & RTS/CTS", "DTR/DSR", "XON/XOFF & DTR/DSR"] ("flow control (0:none)")
              w357 = u16 10 items=["1.0"=10, "1.5"=15, "2.0"=20] ("stop bits (10: 1 bit)")
              n197 = call-poly "VISA Configure Serial Port"("VISA resource name"=w354, "Enable Termination\nChar (T)"=FALSE ("Enable Termination\nChar (T)"), "baud rate (9600)"=w353, "data bits (8)"=u16 8, "parity (0:none)"=enum16{"None", "Odd", "Even", "Mark", "Space"}."None", "stop bits (10: 1 bit)"=w357, "flow control (0:none)"=w358) -> ("VISA resource name out"=w352:refnum<visa-resource-name>, "error out"=w351:errorcluster)  [unwired: 7 in]
              n198 = local read "term"() -> (w364:string)
              n199 = Concatenate Strings(w364, "   MC-BonOMM (" ("string"), w360, ") ... " ("string")) -> (w363:string)
              n200 = Unbundle By Name(w351) -> ("status"=w365:bool)
              n201 = local write "term"(w363) -> ()
              n202 = Not(x=w365) -> (.not. x?=w359:bool)
            }
          }
          n203 = case shown="False" w266 {
            tunnel: w265 -> [w283 w290]
            tunnel: [refnum<visa-resource-name> "-1" ("VISA resource name out") w290] -> w264
            tunnel: [w281 w288] -> w262
            tunnel: w259 -> [w280 w288]
            frame False {
              w282 = FALSE ("Ports Series")
              n204 = local read "term"() -> (w286:string)
              n205 = VISA Close(VISA resource name=w283, error in (no error)=w280) -> (error out=w281:errorcluster)
              n206 = local write "Ports Series"(w282) -> ()
              n207 = Concatenate Strings(w286, "Erreur!\n" ("string")) -> (w285:string)
              n208 = local write "Go on ?"(w282) -> ()
              n209 = local write "term"(w285) -> ()
            }
            frame True {
              n210 = local read "term"() -> (w292:string)
              n211 = Concatenate Strings(w292, "OK!\n" ("string")) -> (w291:string)
              n212 = local write "term"(w291) -> ()
            }
          }
        }
        "Array of VISA refnum" <- w247
        "Serial" <- w246
        "Array of Baud Rates" <- w245
        n213 = local read "term"() -> (w257:string)
        n214 = Concatenate Strings(w257, "Test des ports séries utilisés :\n" ("string")) -> (w258:string)
        n215 = local write "term"(w258) -> ()
        n216 = call <vilib>:"Close Config Data.vi"("error in (no error)"=w251, "refnum"=w253) -> ("error out"=→"config error out":errorcluster)  [unwired: 8 in, 1 out]
      }
      frame #10 {
        w382 = "communications" ("section")
        n217 = local read "Array of Files"() -> (w392:path[])
        n218 = Index Array(array=w392, index=0) -> (element=w391:path)
        n219 = call <vilib>:"Open Config Data.vi"("configuration file path"=w391) -> ("error out"=w383:errorcluster, "refnum"=w384:T3)  [unwired: 8 in, 1 out]
        n220 = local read "term"() -> (w388:string)
        n221 = Concatenate Strings(w388, "Vérification du lien TCP/IP avec TCS ... " ("string")) -> (w389:string)
        n222 = local write "term"(w389) -> ()
        n223 = call-poly <vilib>:"Read Key.vi"("section"=w382, "error in (no error)"=w383, "key"="TCS-IP", "refnum"=w384) -> ("error out"=w385:errorcluster, "value"=w379:string, "refnum out"=w386:T3)  [unwired: 4 in, 1 out]
        n224 = call-poly <vilib>:"Read Key.vi"("section"=w382, "error in (no error)"=w385, "key"="TCS-PN", "refnum"=w386) -> ("error out"=w369:errorcluster, "value"=w378:u32, "refnum out"=w370:T3)  [unwired: 4 in, 1 out]
        n225 = To Unsigned Word Integer(number=w378) -> (unsigned 16bit integer=w377:u16)
        n226 = call <vilib>:"Close Config Data.vi"("error in (no error)"=w369, "refnum"=w370) -> ()  [unwired: 8 in, 2 out]
        n227 = TCP Open Connection(address=w379, remote port or service name=w377, timeout ms (60000)=3000) -> (connection ID=w376:refnum<k5>, error out=w373:errorcluster)  [unwired: 2 in]
        n228 = Unbundle By Name(w373) -> ("status"=w372:bool)
        n229 = Type Cast(type="", x=w376) -> (*(type *) &x=w374:string)
        n230 = Not(x=w372) -> (.not. x?=w367:bool)
        "TCS" <- w367
        n231 = Type Cast(type=refnum<visa-resource-name> "-1" ("Table VRN"), x=w374) -> (*(type *) &x=→"TCS-CommVRN":refnum<visa-resource-name>)
        n232 = case shown="False" w367 {
          selector: w367 -> [w393 _]
          frame False {
            n233 = local write "Go on ?"(w393) -> ()
          }
          frame True {
          }
        }
      }
      frame #11 {
        n234 = local read "TCS"() -> (w394:bool)
        n235 = Select(t="OK!\n" ("string"), s=w394, f="Erreur!\n" ("string")) -> (s? t:f=w397:string)
        n236 = local read "term"() -> (w398:string)
        n237 = Concatenate Strings(w398, w397) -> (w399:string)
        n238 = local write "term"(w399) -> ()
      }
      frame #12 {
        w414 = "communications" ("section")
        n239 = local read "Array of Files"() -> (w421:path[])
        n240 = local read "term"() -> (w424:string)
        n241 = Index Array(array=w421, index=0) -> (element=w420:path)
        n242 = Concatenate Strings(w424, "Vérification du lien avec PRAMMS ... " ("string")) -> (w425:string)
        n243 = local write "term"(w425) -> ()
        n244 = call <vilib>:"Open Config Data.vi"("configuration file path"=w420) -> ("error out"=w415:errorcluster, "refnum"=w416:T3)  [unwired: 8 in, 1 out]
        n245 = call-poly <vilib>:"Read Key.vi"("section"=w414, "error in (no error)"=w415, "key"="PRAMMS-IP", "refnum"=w416) -> ("error out"=w417:errorcluster, "value"=w403:string, "refnum out"=w418:T3)  [unwired: 4 in, 1 out]
        n246 = call-poly <vilib>:"Read Key.vi"("section"=w414, "error in (no error)"=w417, "key"="PRAMMS-PN", "refnum"=w418) -> ("error out"=w406:errorcluster, "value"=w411:u32, "refnum out"=w407:T3)  [unwired: 4 in, 1 out]
        n247 = To Unsigned Word Integer(number=w411) -> (unsigned 16bit integer=w402:u16)
        n248 = call <vilib>:"Close Config Data.vi"("error in (no error)"=w406, "refnum"=w407) -> ()  [unwired: 8 in, 2 out]
        n249 = call "SAOMM-connect.vi"("IP"=w403, "Port"=w402) -> ("connection ID"=w401:refnum<k5>, "Error OUT"=w400:errorcluster)  [unwired: 12 in]
        n250 = Unbundle By Name(w400) -> ("status"=w408:bool)
        n251 = Type Cast(type="", x=w401) -> (*(type *) &x=w409:string)
        n252 = Not(x=w408) -> (.not. x?=w422:bool)
        "PRAMMS" <- w422
        n253 = Type Cast(type=refnum<visa-resource-name> "-1" ("Table VRN"), x=w409) -> (*(type *) &x=→"PRAMMS-CommVRN":refnum<visa-resource-name>)
        n254 = case shown="False" w422 {
          selector: w422 -> [w426 _]
          frame False {
            n255 = local write "Go on ?"(w426) -> ()
          }
          frame True {
          }
        }
      }
      frame #13 {
        n256 = local read "PRAMMS"() -> (w427:bool)
        n257 = Select(t="OK!\n" ("string"), s=w427, f="Erreur!\n" ("string")) -> (s? t:f=w430:string)
        n258 = local read "term"() -> (w431:string)
        n259 = Concatenate Strings(w431, w430) -> (w432:string)
        n260 = local write "term"(w432) -> ()
      }
      frame #14 {
        n261 = flat-sequence {
          tunnel: [w447] -> w441
          tunnel: [w445] -> w440
          tunnel: [w448] -> w438
          tunnel: [w447] -> w437
          tunnel: [w445] -> w434
          tunnel: w441 -> [w467]
          tunnel: w440 -> [w466]
          tunnel: [w465] -> w439
          tunnel: w438 -> [_]
          tunnel: w437 -> [w464]
          tunnel: [w464] -> w436
          tunnel: [w463] -> w435
          tunnel: w434 -> [w462]
          tunnel: [w462] -> w433
          tunnel: w439 -> [w474]
          tunnel: w436 -> [w475]
          tunnel: w435 -> [w471]
          tunnel: w433 -> [w473]
          frame #0 {
            w453 = "communications" ("section")
            n262 = local read "Array of Files"() -> (w444:path[])
            n263 = Index Array(array=w444, index=0) -> (element=w442:path)
            n264 = call <vilib>:"Open Config Data.vi"("configuration file path"=w442) -> ("error out"=w454:errorcluster, "refnum"=w455:T3)  [unwired: 8 in, 1 out]
            n265 = call-poly <vilib>:"Read Key.vi"("section"=w453, "error in (no error)"=w454, "key"="cRIO-PN" ("section"), "refnum"=w455) -> ("error out"=w456:errorcluster, "value"=w446:u32, "refnum out"=w457:T3)  [unwired: 4 in, 1 out]
            n266 = To Unsigned Word Integer(number=w446) -> (unsigned 16bit integer=w445:u16)
            n267 = local read "term"() -> (w459:string)
            n268 = call-poly <vilib>:"Read Key.vi"("section"=w453, "error in (no error)"=w456, "key"="cRIO-IP" ("section"), "refnum"=w457) -> ("error out"=w449:errorcluster, "value"=w447:string, "refnum out"=w450:T3)  [unwired: 4 in, 1 out]
            n269 = Concatenate Strings(w459, "Connexion à la station météo ... " ("string")) -> (w460:string)
            n270 = local write "term"(w460) -> ()
            n271 = call <vilib>:"Close Config Data.vi"("error in (no error)"=w449, "refnum"=w450) -> ("error out"=w448:errorcluster)  [unwired: 8 in, 1 out]
          }
          frame #1 {
            n272 = TCP Open Connection(address=w467, remote port or service name=w466, timeout ms (60000)=3000) -> (connection ID=w463:refnum<k5>, error out=w469:errorcluster)  [unwired: 2 in]
            n273 = Unbundle By Name(w469) -> ("status"=w468:bool)
            n274 = Not(x=w468) -> (.not. x?=w465:bool)
          }
          frame #2 {
            n275 = case shown="False" w474 {
              tunnel: w471 -> [_ _]
              frame False {
                n276 = local read "term"() -> (w478:string)
                n277 = Concatenate Strings(w478, "Erreur!\n" ("string")) -> (w477:string)
                n278 = local write "Go on ?"(FALSE) -> ()
                n279 = local write "term"(w477) -> ()
              }
              frame True {
                n280 = local read "term"() -> (w481:string)
                n281 = Concatenate Strings(w481, "OK!\n" ("string")) -> (w480:string)
                n282 = local write "term"(w480) -> ()
              }
            }
            n283 = TCP Close Connection(connection ID=w471) -> (error out=→"TCP Error":errorcluster)  [unwired: 2 in, 1 out]
            n284 = Bundle("value"=w475, w473, "connection ID"=w471, w474) -> (w472:T4)  [unwired: 1 in]
            n285 = local write "Bundle-Meteo"(w472) -> ()
          }
        }
      }
      frame #15 {
        w506 = "chemins"
        n286 = local read "Array of Files"() -> (w491:path[])
        n287 = Index Array(array=w491, index=0) -> (element=w492:path)
        n288 = call <vilib>:"Open Config Data.vi"("configuration file path"=w492) -> ("error out"=w509:errorcluster, "refnum"=w510:T3)  [unwired: 8 in, 1 out]
        n289 = call-poly <vilib>:"Read Key.vi"("section"=w506, "error in (no error)"=w509, "key"="wgetexec", "refnum"=w510) -> ("error out"=w511:errorcluster, "value"=w488:path, "refnum out"=w512:T3)  [unwired: 4 in, 1 out]
        n290 = flat-sequence {
          tunnel: w488 -> [w538]
          tunnel: [w537] -> w501
          tunnel: [w536] -> w483
          tunnel: w503 -> [w541]
          tunnel: [w540] -> w502
          tunnel: [w539] -> w484
          frame #0 {
            n291 = File/Directory Info(path=w538) -> (error out=w537:errorcluster, resolved path=w536:path)  [unwired: 1 in, 5 out]
          }
          frame #1 {
            n292 = File/Directory Info(path=w541) -> (error out=w540:errorcluster, resolved path=w539:path)  [unwired: 1 in, 5 out]
          }
        }
        n293 = local read "term"() -> (w496:string)
        n294 = Concatenate Strings(w496, "Vérification de l'existence des applications externes ... " ("string")) -> (w497:string)
        n295 = call-poly <vilib>:"Read Key.vi"("section"=w506, "error in (no error)"=w511, "key"="idlexec", "refnum"=w512) -> ("error out"=w507:errorcluster, "value"=w503:path, "refnum out"=w508:T3)  [unwired: 4 in, 1 out]
        n296 = local write "term"(w497) -> ()
        n297 = call <vilib>:"Close Config Data.vi"("error in (no error)"=w507, "refnum"=w508) -> ("error out"=→"error out":errorcluster, "file path"=w489:path)  [unwired: 8 in]
        n298 = Unbundle By Name(w501) -> ("status"=w499:bool)
        n299 = Unbundle By Name(w502) -> ("status"=w500:bool)
        n300 = Not(x=w500) -> (.not. x?=w498:bool)
        n301 = Not(x=w499) -> (.not. x?=w490:bool)
        n302 = local write "IDL"(w498) -> ()
        n303 = local write "wget"(w490) -> ()
        n304 = case shown="True" w490 {
          tunnel: w489 -> [_ w522]
          tunnel: w488 -> [_ w524]
          tunnel: [path "" w521] -> w485
          frame False {
          }
          frame True {
            n305 = local read "Array of Folders"() -> (w519:path[])
            n306 = call "Get_properties.vi"("Keyword"="queuelib" ("Section"), "Section"="chemins", "properties.ini"=w522) -> ("string"=w525:string)  [unwired: 6 in, 2 out]
            n307 = Index Array(array=w519, index=2) -> (element=w518:path)
            n308 = Path To String(path=w524) -> (string=w515:string)
            n309 = Concatenate Strings(w515, " --timeout=5 --tries=1" ("string"), " --http-user=carpe", " --http-password=noctem ", w525) -> (w526:string)
            "concatenated string" <- w526
            n310 = call <vilib>:"System Exec.vi"("run minimized? (F)"=TRUE, "working directory"=w518, "command line"=w526) -> ("error out"=w523:errorcluster, "standard error"=→"standard error":string, "standard output"=→"standard output":string)  [unwired: 5 in, 1 out]
            n311 = case shown="No Error" w523 {
              tunnel: w518 -> [w534 _]
              tunnel: [w532 path ""] -> w521
              frame No Error {
                n312 = Build Path(base path=w534, name or relative path="table_technicien.dat") -> (appended path=w532:path)
              }
              frame Error {
              }
            }
          }
        }
        n313 = local read "Array of Files"() -> (w486:path[])
        n314 = Build Array (concatenate)(w486, w485, w484, w483) -> (w487:path[])
        n315 = local write "Array of Files"(w487) -> ()
      }
      frame #16 {
        n316 = local read "wget"() -> (w548:bool)
        n317 = local read "IDL"() -> (w549:bool)
        n318 = And(x=w549, y=w548) -> (x .and. y?=w542:bool)
        n319 = Select(t="OK!\n" ("string"), s=w542, f="Erreur!\n" ("string")) -> (s? t:f=w543:string)
        n320 = case shown="False" w542 {
          selector: w542 -> [w550 _]
          frame False {
            n321 = local write "Go on ?"(w550) -> ()
          }
          frame True {
          }
        }
        n322 = local read "term"() -> (w547:string)
        n323 = Concatenate Strings(w547, w543) -> (w546:string)
        n324 = local write "term"(w546) -> ()
      }
      frame #17 {
        # "VIs requierant une référence ou dont la face avant doit être caché"
        n325 = for {
          tunnel: string[] ["GUI\\CameraTuning.vi", "GUI\\Mode sync(pop-up).vi", "GUI\\InstrChoice.vi"] -> [w577] mode=indexing
          tunnel: [w572] -> w552 mode=indexing
          tunnel: [w571] -> w551 mode=indexing
          i -> [w566]
          n326 = local read "Array of Folders"() -> (w570:path[])
          n327 = Index Array(array=w570, index=4) -> (element=w569:path)
          n328 = Build Path(base path=w569, name or relative path=w577) -> (appended path=w576:path)
          n329 = Open VI Reference(vi path=w576) -> (vi reference=w567:refnum<vi>, error out=w565:errorcluster)  [unwired: 5 in]
          n330 = case shown="0" w566 {
            tunnel: w567 -> [_ w579 _ _]
            tunnel: w565 -> [_ w578 _ _]
            frame -1, Default {
            }
            frame 0 {
              n331 = case shown="No Error" w578 {
                tunnel: w579 -> [w580 _]
                frame No Error {
                  n332 = global write "Globals.vi" "CameraTuning VI Refnum"(w580) -> ()
                }
                frame Error {
                }
              }
            }
            frame 1 {
            }
            frame 2 {
            }
          }
          n333 = property class="VI"(reference=w567, error in=w565) -> (reference out=w574:refnum<vi>, error out=w573:errorcluster, "Front Panel.Open"=w575:bool)
          n334 = case shown="True" w575 {
            tunnel: w574 -> [w582 w587]
            tunnel: [w582 w586] -> w572
            tunnel: w573 -> [w581 w584]
            tunnel: [w581 w583] -> w571
            frame False {
            }
            frame True {
              n335 = property class="VI"(reference=w587, error in=w584, "Front Panel.Open"=FALSE) -> (reference out=w586:refnum<vi>, error out=w583:errorcluster)
            }
          }
        }
        n336 = local read "term"() -> (w554:string)
        n337 = Concatenate Strings(w554, "Vérification de l'état des sous-vis ... " ("string")) -> (w555:string)
        n338 = local write "term"(w555) -> ()
        n339 = flat-sequence {
          tunnel: w552 -> [_]
          tunnel: w551 -> [w560]
          frame #0 {
            n340 = for {
              tunnel: w560 -> [w564] mode=indexing
              tunnel: [w563] -> w559 mode=indexing
              n341 = Unbundle By Name(w564) -> ("status"=w563:bool)
            }
            n342 = Boolean Array To Number(Boolean array=w559) -> (number=w558:u32)
            n343 = Wait (ms)(milliseconds to wait=u32 500) -> ()  [unwired: 1 out]
            n344 = Greater Than 0?(x=w558) -> (x > 0?=w557:bool)
            n345 = case shown="True" w557 {
              frame False {
              }
              frame True {
                w562 = FALSE
                n346 = local write "Go on ?"(w562) -> ()
                n347 = local write "SubVIs"(w562) -> ()
              }
            }
          }
        }
      }
      frame #18 {
        n348 = local read "SubVIs"() -> (w588:bool)
        n349 = Select(t="OK!\n" ("string"), s=w588, f="Erreur!\n" ("string")) -> (s? t:f=w591:string)
        n350 = local read "term"() -> (w592:string)
        n351 = Concatenate Strings(w592, w591) -> (w593:string)
        n352 = local write "term"(w593) -> ()
      }
      frame #19 {
        # "Mettre à la fin pour recommencer tout ..."
        n353 = local read "Go on ?"() -> (w597:bool)
        n354 = case shown="False" w597 {
          tunnel: [w627 FALSE ("true")] -> w598
          frame False {
            w626 = T2."Enabled" ("Disabled")
            n355 = One Button Dialog(message="Une ou plusieurs erreurs se sont produites lors de l'initialisation.\nVous pouvez annuler l'ouverture du programme, recommencez l'initialisation ou ignorer les erreurs.\n\nCependant, si vous ignorez les erreurs, il se peut que \ncertaines fonctionnalités ne soient pas disponibles") -> (true=w627:bool)  [unwired: 1 in]
            n356 = property on="cancel" class="Bool"("DisabledEnum"=w626) -> ()  [unwired: 2 in, 2 out]
            n357 = property on="ignore" class="Bool"("DisabledEnum"=w626) -> ()  [unwired: 2 in, 2 out]
            n358 = property on="restart" class="Bool"("DisabledEnum"=w626) -> ()  [unwired: 2 in, 2 out]
          }
          frame True {
          }
        }
        n359 = local read "term"() -> (w594:string)
        n360 = case shown="True" w598 {
          tunnel: [u32 0 w608] -> w596
          tunnel: w594 -> [_ w607]
          frame False {
            (unwired) TRUE
          }
          frame True {
            n361 = while {
              tunnel: [w619] -> w608
              tunnel: w607 -> [w615]
              i -> [w618]
              stop <- w621 stop-if-true
              n362 = Build Array("cancel", "restart", "ignore") -> (w620:bool[])
              n363 = Quotient & Remainder(x=w618, y=10) -> (x-y*floor(x/y)=w611:i32)  [unwired: 1 out]
              n364 = Boolean Array To Number(Boolean array=w620) -> (number=w619:u32)
              n365 = Less?(x=w611, y=6) -> (x < y?=w610:bool)
              n366 = Wait (ms)(milliseconds to wait=u32 100) -> ()  [unwired: 1 out]
              n367 = Greater Than 0?(x=w619) -> (x > 0?=w621:bool)
              n368 = Select(t="\nEn attente de la réponse de l'usagé ..." ("string"), s=w610, f="") -> (s? t:f=w613:string)
              n369 = Concatenate Strings(w615, w613) -> (w614:string)
              n370 = local write "term"(w614) -> ()
            }
          }
        }
        n371 = case shown="1" w596 {
          tunnel: [TRUE TRUE FALSE TRUE] -> w595
          frame 0, Default {
          }
          frame 1 {
            n372 = local write "Go on ?"(FALSE ("Go on ?")) -> ()
          }
          frame 2 {
            n373 = local write "Go on ?"(FALSE ("Go on ?")) -> ()
          }
          frame 4 {
            n374 = local write "Go on ?"(TRUE ("Go on ?")) -> ()
          }
        }
      }
      frame #20 {
        n375 = local read "Go on ?"() -> (w631:bool)
        n376 = case shown="True" w631 {
          tunnel: w630 -> [_ w632]
          frame False {
          }
          frame True {
            n377 = flat-sequence {
              tunnel: w632 -> [w633]
              frame #0 {
                n378 = Concatenate Strings(w633, "\nVérifications complétées\nBonne Nuit !!!" ("string")) -> (w635:string)
                n379 = local write "term"(w635) -> ()
              }
              frame #1 {
                n380 = Wait (ms)(milliseconds to wait=u32 666) -> ()  [unwired: 1 out]
              }
            }
          }
        }
      }
    }
  }
  n381 = disable-structure shown="Disabled" {
    frame Disabled {
      n382 = flat-sequence {
        tunnel: w656 -> [w659]
        tunnel: [w659] -> w637
        frame #0 {
          n383 = Wait (ms)(milliseconds to wait=u32 500) -> ()  [unwired: 1 out]
        }
      }
      n384 = call "MC-BonOMM_talker.vi"("MC-BonOMM VRN"=w637, "Commande"="m", "byte count"=u32 1, "Timeout (ms)"=3000, "answer=command?"=FALSE) -> ("Answer"=w639:string, "ok ?"=w640:bool)
      n385 = VISA Write(write buffer="r" ("Commande")) -> (VISA resource name=w654:refnum<visa-resource-name>, error in (no error)=w655:errorcluster, VISA resource name out=w652:refnum<visa-resource-name>)  [unwired: 2 out]
      n386 = property class="Instr"(reference=w652) -> (reference out=w651:refnum<visa-resource-name>, "Serial Settings:Number of Bytes at Serial Port"=w650:u32)  [unwired: 1 in, 1 out]
      n387 = Equal?(x="f", y=w639) -> (x = y?=w644:bool)
      n388 = Equal?(x=w639, y="x") -> (x = y?=w645:bool)
      n389 = Or(x=w644, y=w645) -> (x .or. y?=w641:bool)
      n390 = And(x=w641, y=w640) -> (x .and. y?=w638:bool)
      n391 = VISA Read(VISA resource name=w651, byte count=w650) -> (VISA resource name out=w656:refnum<visa-resource-name>)  [unwired: 1 in, 3 out]
      n392 = case shown="True" w638 {
        tunnel: [w660 w674] -> w657
        tunnel: w656 -> [_ w665]
        frame False {
          n393 = Two Button Dialog(message="MC-BonOMM n'a pas été détecté !\nSouhaitez-vous recommencer l'initalisation ?", 1:"NON" ("F button name (\"Cancel\")"), 2:"OUI" ("T button name (\"OK\")")) -> (T button?=w661:bool)
          n394 = Not(x=w661) -> (.not. x?=w660:bool)
        }
        frame True {
          n395 = call <vilib>:"Three Button Dialog.vi"("Allow user to close window? (TRUE)"=FALSE, "Justify Message (Left)"=enum16{"Left", "Center", "Right"}."Center", "Right Button Text (\"Cancel\")"="Foyer ST-133" ("F button name (\"Cancel\")"), "Center Button Text (\"No\")"="RàF (PANO-II)" ("F button name (\"Cancel\")"), "Left Button Text (\"Yes\")"="RàF (BonOMM)" ("T button name (\"OK\")"), "message"="MC-BonOMM a été détecté !\nQuel mode souhaité vous utiliser ?") -> ("Which Button?"=w667:T5)  [unwired: 5 in]
          n396 = case shown="\"Left Button\", Default" w667 {
            tunnel: ["o" "x" "f"] -> w666
            frame "Center Button" {
            }
            frame "Right Button" {
            }
            frame "Left Button", Default {
            }
          }
          n397 = call "MC-BonOMM_talker.vi"("MC-BonOMM VRN"=w665, "Commande"=w666, "Timeout (ms)"=1000, "answer=command?"=TRUE) -> ("ok ?"=w674:bool)  [unwired: 1 in, 1 out]
        }
      }
    }
    frame Enabled {
    }
  }
